vi "DtCreateDOutChan.vi"(5 "Board Name":string, 9 "Port Number":u32, 11 "error in (no error)":errorcluster) -> (4 "Task out":i32, 15 "error out":errorcluster)   [LabVIEW 2016]
doc: "Creates one or more virtual digital output ports that you can update. LV-Link automatically configures the digital output port with the default resolution supported by the subsystem.\n\nSome DT-Open Layers devices have bidirectional digital ports. For these ports, calling this VI configures the digital port as an output. If you then try to call the Digital Input instance of this VI on the same port, an error will result. To reconfigure the port as an input, you must first stop the digital output task by calling the DtOLStop VI, and then call the Digital Input instance of this VI.\n\nOnce you have created a virtual digital output port, you can start the task and update the port using the DtOLWrite (Write Single Channel - Single Sample) VI."
uses:
  <userlib>/LV-Link3/DtLvLink.lvlib
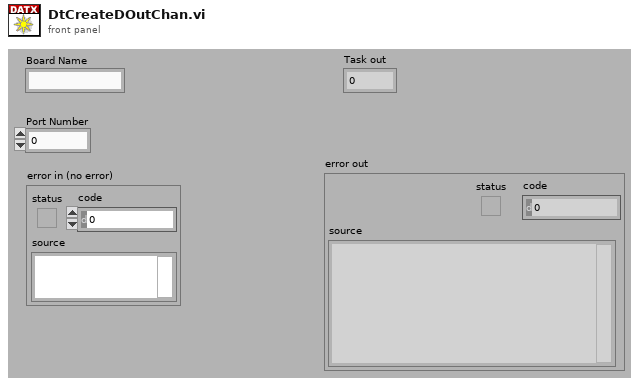
[diagram p1: front panel]
types:
  T1 = enum32{"AnalogInput", "AnalogOutput", "DigitalInput", "DigitalOutput", "Quadrature", "CounterTimer"}
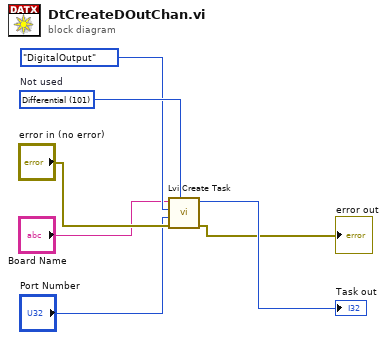
[diagram p0: block diagram]
diagram:
  w7 = 101 items=["SingleEnded"=100, "Differential"=101]  # Not used
  n1 = call <userlib>:"Lvi Create Task.vi"("SEorDiff"=w7, "error in (no error)"="error in (no error)", "SubSysIndex"="Port Number", "ChanType"=T1."DigitalOutput", "BoardName"="Board Name") -> ("error out"=→"error out":errorcluster, "TaskRef"=→"Task out":i32)  [unwired: 4 in, 1 out]
